vi "PicoHandsOnExample.vi"() -> ()   [LabVIEW 2022 SP3, in "HandsOnPi2040.lvlib"]
uses:
  <instrlib>/HandsOnPi2040/HandsOnPi2040.lvlib
  <instrlib>/HandsOnPi2040/Public/DigIns.ctl
  <instrlib>/HandsOnPi2040/Public/AnaIns.ctl
  <instrlib>/HandsOnPi2040/cti-drivers-lv-visa-main/CTI-Visa/Identity.ctl
  <instrlib>/HandsOnPi2040/Public/DigOuts.ctl
  <instrlib>/HandsOnPi2040/Public/AOs.ctl
  <instrlib>/HandsOnPi2040/Public/PWMSettings.ctl
  <instrlib>/HandsOnPi2040/cti-drivers-lv-visa-main/CTI-Visa/CTI-Visa.lvlib
panel:
  in  "Frequency":sgl(slide) scale=10.0..500000.0
  in  "Duty":sgl(slide) scale=0.0..1.0
  out "Identity":T1
  out "LoopIndex":i32
  in  "Digital Output":T2(ring)=enum."DO1"
  in  "DOBEEP":bool
  in  "DO4":bool
  in  "DO3":bool
  in  "DO2":bool
  out "AnInValue":u16(graph)
  in  "Analog Inputs":T3=enum."AI1"
  out "DIStatus":bool
  in  "Digital Inputs":T4=enum."DI1"
  out "DOStatus":bool
  in  "DO1":bool
  in  "VISA resource name":refnum<visa-resource-name>="TCPIP0::192.168.10.207::6430::SOCKET"
  out "error out":errorcluster
  in  "stop":bool
  # "READ"
  # "WRITE"
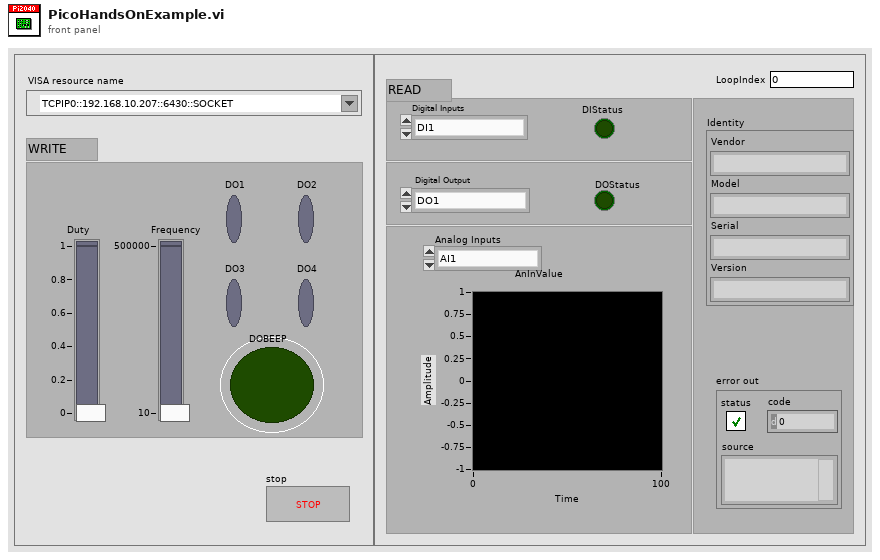
[diagram p1: front panel]
types:
  T1 = typedef "CTI-Visa.lvlib/Identity.ctl" = cluster{"Vendor":string, "Model":string, "Serial":string, "Version":string}
  T2 = enum16{"No DO - Error", "DO1", "DO2", "DO3", "DO4", "BEEP"}
  T3 = typedef "HandsOnPi2040.lvlib/AnaIns.ctl" = enum16{"No AI - Error", "AI1", "AI2"}
  T4 = typedef "HandsOnPi2040.lvlib/DigIns.ctl" = enum16{"No DI - Error", "DI1", "DI2", "DI3", "DI4"}
  T5 = typedef "HandsOnPi2040.lvlib/DigOuts.ctl" = enum16{"No DO - Error", "DO1", "DO2", "DO3", "DO4", "BEEP"}
  T6 = typedef "HandsOnPi2040.lvlib/PWMSettings.ctl" = cluster{"Duty":sgl, "Frequency":sgl}
  T7 = typedef "HandsOnPi2040.lvlib/AOs.ctl" = enum16{"No AO - Error", "AO1"}
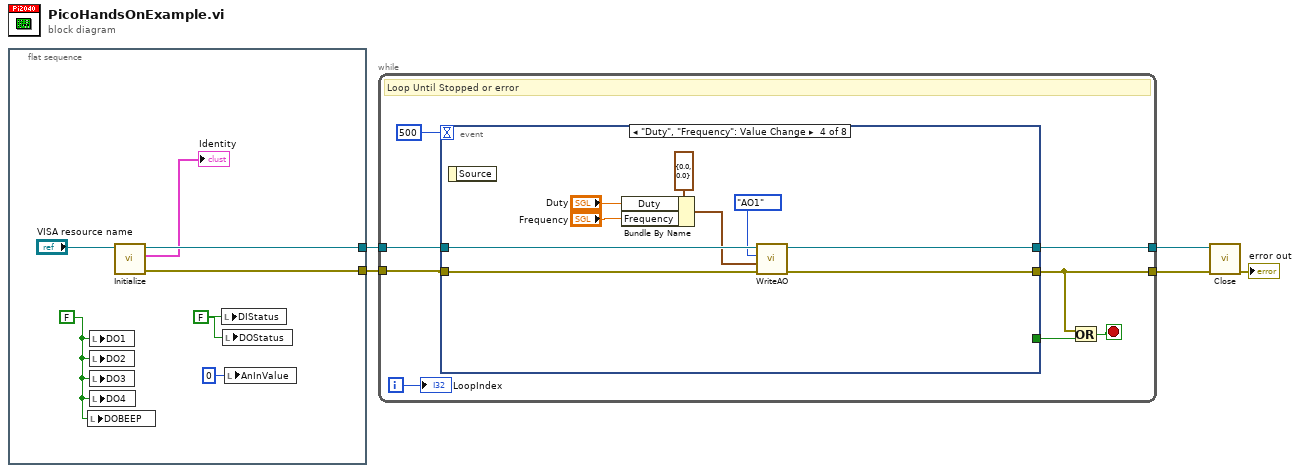
[diagram p0: block diagram]
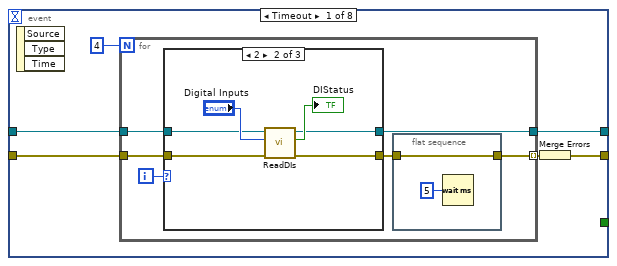
[diagram p2: hidden frame]
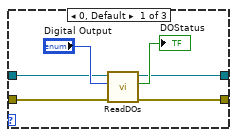
[diagram p3: hidden frame]
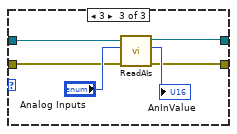
[diagram p4: hidden frame]
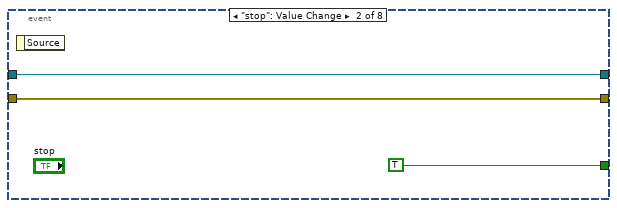
[diagram p5: hidden frame]
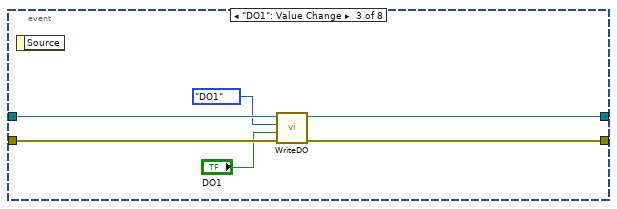
[diagram p6: hidden frame]
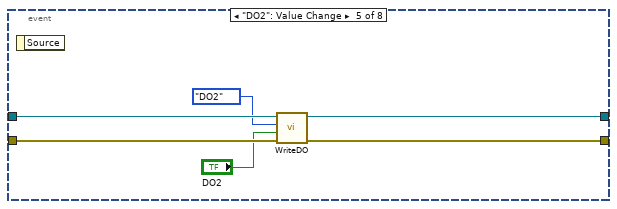
[diagram p7: hidden frame]
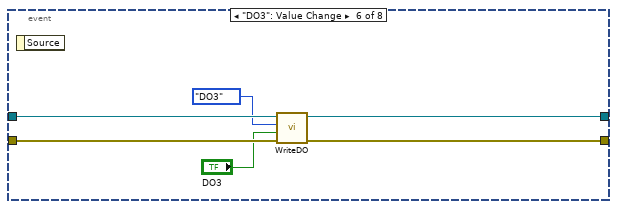
[diagram p8: hidden frame]
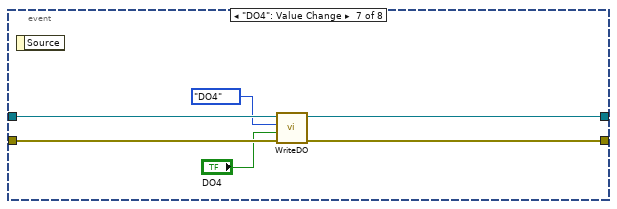
[diagram p9: hidden frame]
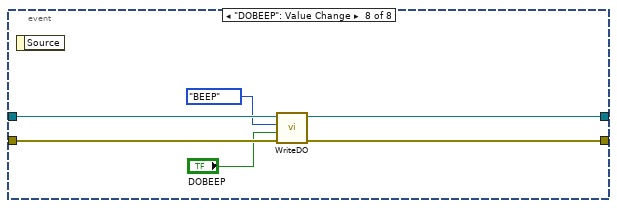
[diagram p10: hidden frame]
diagram:
  n1 = flat-sequence {
    tunnel: [w11] -> w2
    tunnel: [w10] -> w1
    frame #0 {
      w8 = FALSE ("WriteAnOut")
      w9 = FALSE ("WriteAnOut")
      n2 = local write "DOBEEP"(w9) -> ()
      n3 = local write "DO1"(w9) -> ()
      n4 = local write "DO2"(w9) -> ()
      n5 = local write "DO3"(w9) -> ()
      n6 = local write "DO4"(w9) -> ()
      n7 = call <instrlib>:"Initialize.vi"("VISA resource name"="VISA resource name") -> ("error out"=w10:errorcluster, "Identity"=→"Identity":T1, "VISA resource name out"=w11:refnum<visa-resource-name>)  [unwired: 8 in]
      n8 = local write "DIStatus"(w8) -> ()
      n9 = local write "DOStatus"(w8) -> ()
      n10 = local write "AnInValue"(u16 0 ("AnInValue")) -> ()
    }
  }
  n11 = while {
    tunnel: [w15] -> w5
    tunnel: w2 -> [w20]
    tunnel: [w19] -> w3
    tunnel: w1 -> [w17]
    i -> [w16]
    stop <- w13 stop-if-true
    # "Loop Until Stopped or error"
    n12 = event shown="[3] \"Duty\", \"Frequency\": Value Change" {
      selector: _ -> [_ _ _ _ _ _ _ _]
      dyn-events: _ -> [_ _ _ _ _ _ _ _]
      timeout: 500 -> [_ _ _ _ _ _ _ _]
      tunnel: [_ TRUE _ _ _ _ _ _] -> w14
      tunnel: [w24 w53 w61 w67 w76 w82 w88 w94] -> w15
      tunnel: w17 -> [w26 w53 w60 w69 w75 w81 w87 w93]
      tunnel: w20 -> [w23 w54 w59 w70 w74 w80 w86 w92]
      tunnel: [w22 w54 w58 w68 w73 w79 w85 w91] -> w19
      event Timeout {
        n13 = event-data() -> ()  [unwired: 1 in, 3 out]
        n14 = for {
          N: 4 -> [_]
          tunnel: w26 -> [w31]
          tunnel: [w27] -> w25 mode=indexing
          tunnel: w23 -> [w30]
          tunnel: [w29] -> w22
          i -> [w32]
          n15 = case shown="2" w32 {
            tunnel: w31 -> [w38 w43 w49]
            tunnel: [w37 w41 w47] -> w28
            tunnel: w30 -> [w36 w44 w50]
            tunnel: [w35 w42 w48] -> w29
            frame 0, Default {
              n16 = call <instrlib>:"ReadDOs.vi"("error in (no error)"=w38, "Output"="Digital Output", "VISA resource name"=w36) -> ("error out"=w37:errorcluster, "DOStatus"=→"DOStatus":bool, "VISA resource name out"=w35:refnum<visa-resource-name>)  [unwired: 6 in]
            }
            frame 2 {
              n17 = call <instrlib>:"ReadDIs.vi"("error in (no error)"=w43, "Digital Inputs"="Digital Inputs", "VISA resource name"=w44) -> ("error out"=w41:errorcluster, "DIStatus"=→"DIStatus":bool, "VISA resource name out"=w42:refnum<visa-resource-name>)  [unwired: 6 in]
            }
            frame 3 {
              n18 = call <instrlib>:"ReadAIs.vi"("error in (no error)"=w49, "Analog Inputs"="Analog Inputs", "VISA resource name"=w50) -> ("error out"=w47:errorcluster, "Value"=→"AnInValue":u16, "VISA resource name out"=w48:refnum<visa-resource-name>)  [unwired: 6 in]
            }
          }
          n19 = flat-sequence {
            tunnel: w28 -> [w34]
            tunnel: [w34] -> w27
            frame #0 {
              n20 = Wait (ms)(milliseconds to wait=u32 5) -> ()  [unwired: 1 out]
            }
          }
        }
        n21 = Merge Errors(w25) -> (w24:errorcluster)
      }
      event "stop": Value Change {
        n22 = event-data() -> ()  [unwired: 1 in, 1 out]
      }
      event "DO1": Value Change {
        n23 = event-data() -> ()  [unwired: 1 in, 1 out]
        n24 = call <instrlib>:"WriteDO.vi"("error in (no error)"=w60, "DO Value (True)"="DO1", "Output"=DigOuts."DO1" ("Write Digital Output"), "VISA resource name"=w59) -> ("error out"=w61:errorcluster, "VISA resource name out"=w58:refnum<visa-resource-name>)  [unwired: 6 in]
      }
      event "Duty", "Frequency": Value Change {
        n25 = event-data() -> ()  [unwired: 1 in, 1 out]
        n26 = Bundle By Name(cluster=T6 {"Duty"=0.0, "Frequency"=0.0} ("PWM Settings"), "Duty"="Duty", "Frequency"="Frequency") -> (w64:T6)
        n27 = call <instrlib>:"WriteAO.vi"("error in (no error)"=w69, "PWM Settings"=w64, "Analog Output"=AOs."AO1", "VISA resource name"=w70) -> ("error out"=w67:errorcluster, "VISA resource name out"=w68:refnum<visa-resource-name>)  [unwired: 6 in]
      }
      event "DO2": Value Change {
        n28 = event-data() -> ()  [unwired: 1 in, 1 out]
        n29 = call <instrlib>:"WriteDO.vi"("error in (no error)"=w75, "DO Value (True)"="DO2", "Output"=DigOuts."DO2" ("Write Digital Output"), "VISA resource name"=w74) -> ("error out"=w76:errorcluster, "VISA resource name out"=w73:refnum<visa-resource-name>)  [unwired: 6 in]
      }
      event "DO3": Value Change {
        n30 = event-data() -> ()  [unwired: 1 in, 1 out]
        n31 = call <instrlib>:"WriteDO.vi"("error in (no error)"=w81, "DO Value (True)"="DO3", "Output"=DigOuts."DO3" ("Write Digital Output"), "VISA resource name"=w80) -> ("error out"=w82:errorcluster, "VISA resource name out"=w79:refnum<visa-resource-name>)  [unwired: 6 in]
      }
      event "DO4": Value Change {
        n32 = event-data() -> ()  [unwired: 1 in, 1 out]
        n33 = call <instrlib>:"WriteDO.vi"("error in (no error)"=w87, "DO Value (True)"="DO4", "Output"=DigOuts."DO4" ("Write Digital Output"), "VISA resource name"=w86) -> ("error out"=w88:errorcluster, "VISA resource name out"=w85:refnum<visa-resource-name>)  [unwired: 6 in]
      }
      event "DOBEEP": Value Change {
        n34 = event-data() -> ()  [unwired: 1 in, 1 out]
        n35 = call <instrlib>:"WriteDO.vi"("error in (no error)"=w93, "DO Value (True)"="DOBEEP", "Output"=DigOuts."BEEP" ("Write Digital Output"), "VISA resource name"=w92) -> ("error out"=w94:errorcluster, "VISA resource name out"=w91:refnum<visa-resource-name>)  [unwired: 6 in]
      }
    }
    n36 = Or(x=w15, y=w14) -> (x .or. y?=w13:bool)
    "LoopIndex" <- w16
  }
  n37 = call <instrlib>:"Close.vi"("error in (no error)"=w5, "VISA resource name"=w3) -> ("error out"=→"error out":errorcluster)  [unwired: 9 in]
